vi "simple.vi"() -> ()   [LabVIEW 2013]
uses:
  simple_states.ctl
panel:
  in  "Long Task":bool
  in  "Submit":bool
  in  "Operation":T1=enum."Reverse"
  out "Last Operation":T1=enum."Reverse"
  out "Output":string
  in  "Input":string
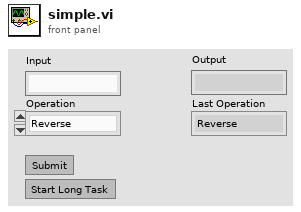
[diagram p1: front panel]
types:
  T1 = typedef "simple_states.ctl" = enum16{"Long Task", "Reverse", "Remove White", "All Lower", "All Upper"}
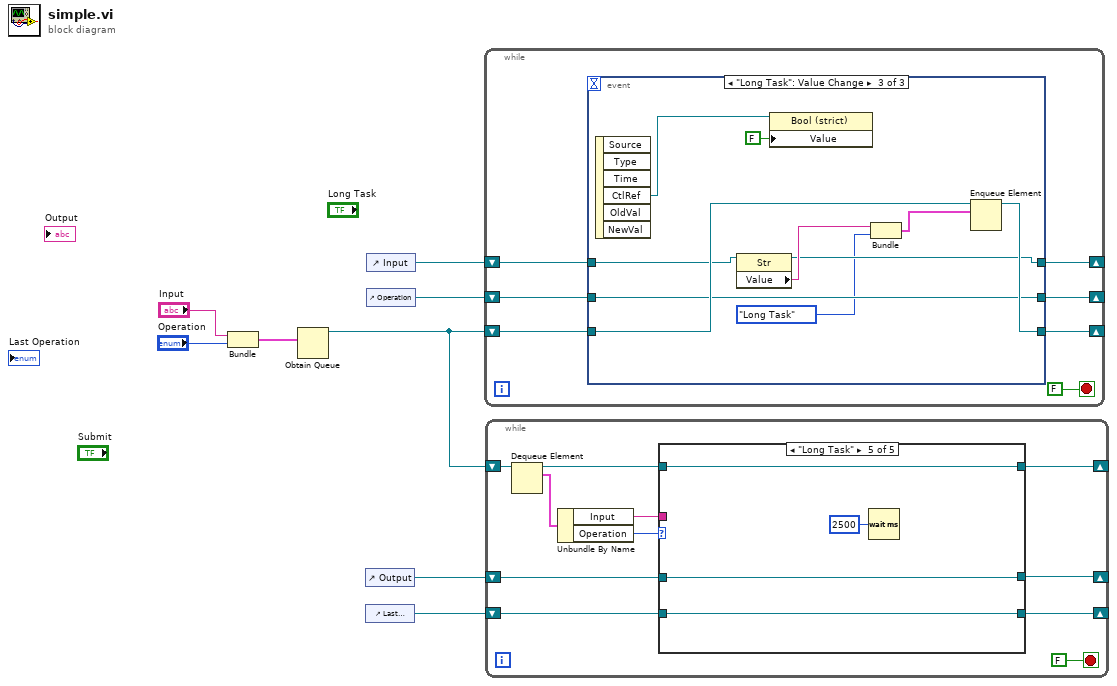
[diagram p0: block diagram]
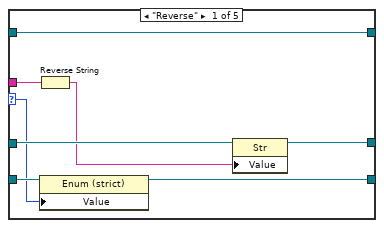
[diagram p2: hidden frame]
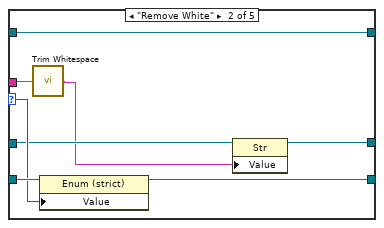
[diagram p3: hidden frame]
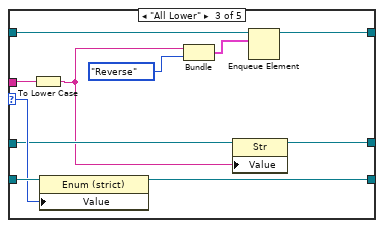
[diagram p4: hidden frame]
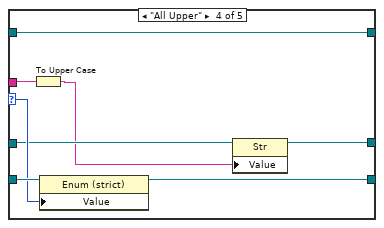
[diagram p5: hidden frame]
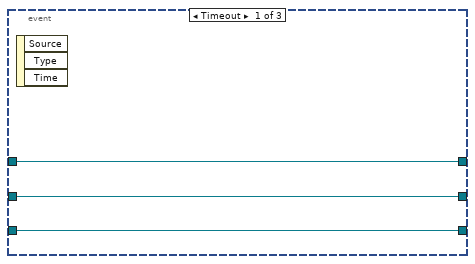
[diagram p6: hidden frame]
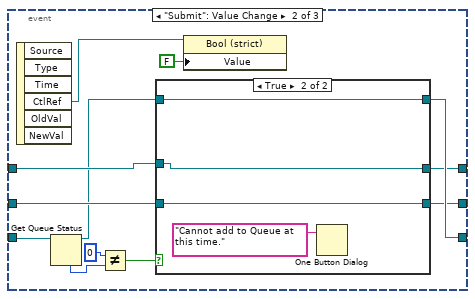
[diagram p7: hidden frame]
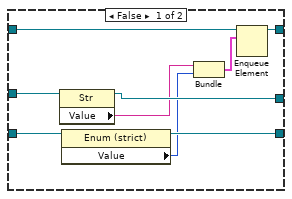
[diagram p8: hidden frame]
diagram:
  n1 = Bundle("Input"="Input", "Operation"="Operation") -> (w6:cluster{"Input":string, "Operation":T1})  [unwired: 1 in]
  n2 = Obtain Queue(element data type=w6) -> (queue out=w8:refnum<queue>)  [unwired: 4 in, 2 out]
  n3 = control-ref of="Output"() -> (w5:refnum<vi>)
  n4 = control-ref of="Last Operation"() -> (w4:refnum<vi>)
  n5 = control-ref of="Input"() -> (w3:refnum<vi>)
  n6 = control-ref of="Operation"() -> (w2:refnum<vi>)
  n7 = while {
    shift-right: [w14] -> _
    shift-left: w8 -> [w15]
    shift-right: [w10] -> _
    shift-left: w3 -> [w12]
    shift-right: [w11] -> _
    shift-left: w2 -> [w13]
    stop <- FALSE stop-if-true
    n8 = event shown="[2] \"Long Task\": Value Change" {
      selector: _ -> [_ _ _]
      dyn-events: _ -> [_ _ _]
      timeout: _ -> [_ _ _]
      tunnel: w15 -> [w16 w23 w51]
      tunnel: [w16 w30 w50] -> w14
      tunnel: w13 -> [w17 w29 w45]
      tunnel: w12 -> [w18 w28 w49]
      tunnel: [w17 w27 w45] -> w11
      tunnel: [w18 w26 w46] -> w10
      event Timeout {
        n9 = event-data() -> ()  [unwired: 1 in, 3 out]
      }
      event "Submit": Value Change {
        n10 = event-data() -> ("CtlRef"=w25:refnum<vi>)  [unwired: 1 in, 5 out]
        n11 = Get Queue Status(queue=w23) -> (queue out=w19:refnum<queue>, # elements in queue=w22:i32)  [unwired: 2 in, 6 out]
        n12 = Not Equal?(x=0, y=w22) -> (x != y?=w20:bool)
        n13 = case shown="True" w20 {
          tunnel: [w39 w43] -> w30
          tunnel: w29 -> [w38 w41]
          tunnel: w28 -> [w37 w42]
          tunnel: [w36 w41] -> w27
          tunnel: [w35 w42] -> w26
          tunnel: w19 -> [w31 w43]
          frame False {
            n14 = property class="Str"(reference=w37) -> (reference out=w35:refnum<vi>, "Value"=w33:string)  [unwired: 1 in, 1 out]
            n15 = property class="Enum (strict)"(reference=w38) -> (reference out=w36:refnum<vi>, "Value"=w34:T1)  [unwired: 1 in, 1 out]
            n16 = Bundle("Value"=w33, "Value"=w34) -> (w32:cluster{"Value":string, "Value":T1})  [unwired: 1 in]
            n17 = Enqueue Element(queue=w31, element=w32) -> (queue out=w39:refnum<queue>)  [unwired: 2 in, 2 out]
          }
          frame True {
            n18 = One Button Dialog(message="Cannot add to Queue at this time.") -> ()  [unwired: 1 in, 1 out]
          }
        }
        n19 = property class="Bool (strict)"(reference=w25, "Value"=FALSE) -> ()  [unwired: 1 in, 2 out]
      }
      event "Long Task": Value Change {
        n20 = event-data() -> ("CtlRef"=w53:refnum<vi>)  [unwired: 1 in, 5 out]
        n21 = property class="Str"(reference=w49) -> (reference out=w46:refnum<vi>, "Value"=w48:string)  [unwired: 1 in, 1 out]
        n22 = property class="Bool (strict)"(reference=w53, "Value"=FALSE) -> ()  [unwired: 1 in, 2 out]
        n23 = Bundle("Value"=w48, "Operation"=simple_states."Long Task") -> (w47:cluster{"Value":string, "Operation":T1})  [unwired: 1 in]
        n24 = Enqueue Element(queue=w51, element=w47) -> (queue out=w50:refnum<queue>)  [unwired: 2 in, 2 out]
      }
    }
  }
  n25 = while {
    shift-right: [w54] -> _
    shift-left: w8 -> [w64]
    shift-right: [w57] -> _
    shift-left: w5 -> [w60]
    shift-right: [w58] -> _
    shift-left: w4 -> [w59]
    stop <- FALSE stop-if-true
    n26 = Dequeue Element(queue=w64) -> (queue out=w55:refnum<queue>, element=w63:cluster{"Input":string, "Operation":T1})  [unwired: 2 in, 2 out]
    n27 = Unbundle By Name(w63) -> ("Input"=w61:string, "Operation"=w62:T1)
    n28 = case shown="\"Long Task\"" w62 {
      selector: w62 -> [w66 w79 w90 w98 _]
      tunnel: w61 -> [w68 w75 w86 w94 _]
      tunnel: w60 -> [w69 w76 w87 w95 w102]
      tunnel: w59 -> [w72 w80 w91 w99 w101]
      tunnel: [w71 w78 w89 w97 w101] -> w58
      tunnel: [w70 w77 w88 w96 w102] -> w57
      tunnel: w55 -> [w65 w73 w85 w92 w100]
      tunnel: [w65 w73 w84 w92 w100] -> w54
      frame "Reverse" {
        n29 = Reverse String(1:w68) -> (0:w67:string)
        n30 = property class="Enum (strict)"(reference=w72, "Value"=w66) -> (reference out=w71:refnum<vi>)  [unwired: 1 in, 1 out]
        n31 = property class="Str"(reference=w69, "Value"=w67) -> (reference out=w70:refnum<vi>)  [unwired: 1 in, 1 out]
      }
      frame "Remove White" {
        n32 = call <vilib>:"Trim Whitespace.vi"("string"=w75) -> ("trimmed string"=w74:string)  [unwired: 1 in]
        n33 = property class="Enum (strict)"(reference=w80, "Value"=w79) -> (reference out=w78:refnum<vi>)  [unwired: 1 in, 1 out]
        n34 = property class="Str"(reference=w76, "Value"=w74) -> (reference out=w77:refnum<vi>)  [unwired: 1 in, 1 out]
      }
      frame "All Lower" {
        n35 = To Lower Case(string=w86) -> (all lower case string=w81:string)
        n36 = property class="Enum (strict)"(reference=w91, "Value"=w90) -> (reference out=w89:refnum<vi>)  [unwired: 1 in, 1 out]
        n37 = Bundle(w81, "Operation"=simple_states."Reverse") -> (w83:cluster{string, "Operation":T1})  [unwired: 1 in]
        n38 = property class="Str"(reference=w87, "Value"=w81) -> (reference out=w88:refnum<vi>)  [unwired: 1 in, 1 out]
        n39 = Enqueue Element(queue=w85, element=w83) -> (queue out=w84:refnum<queue>)  [unwired: 2 in, 2 out]
      }
      frame "All Upper" {
        n40 = To Upper Case(1:w94) -> (0:w93:string)
        n41 = property class="Enum (strict)"(reference=w99, "Value"=w98) -> (reference out=w97:refnum<vi>)  [unwired: 1 in, 1 out]
        n42 = property class="Str"(reference=w95, "Value"=w93) -> (reference out=w96:refnum<vi>)  [unwired: 1 in, 1 out]
      }
      frame "Long Task" {
        n43 = Wait (ms)(milliseconds to wait=u32 2500) -> ()  [unwired: 1 out]
      }
    }
  }
